vi "h.CONST.physics.vi"() -> ()   [LabVIEW 2016, in "h.Library.lvlib"]
doc: "This global contains various physical constants used by Hyperion instruments."
uses:
  h.Library.lvlib
panel:
  in  "SpeedOfLight(m/s)":dbl=299792458.0 format="%#_20f"
  # "Hyperion Physics Constants"
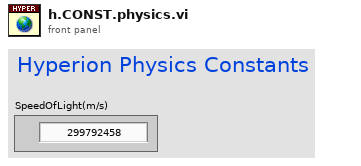
[diagram p1: front panel]
diagram:
